vi "LX-runtime.vi"(11 "Start Time 2":u32) -> (3 "运行时间 2":dbl)   [LabVIEW 2017]
panel:
  out "Start Time":u32
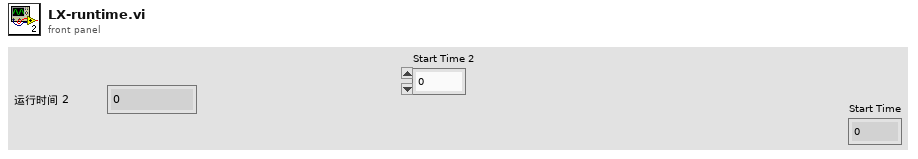
[diagram p1: front panel]
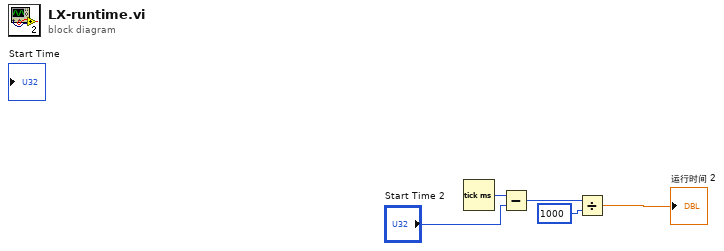
[diagram p0: block diagram]
diagram:
  n1 = Tick Count (ms)() -> (millisecond timer value=w4:u32)
  n2 = Subtract(x=w4, y="Start Time 2") -> (x-y=w5:u32)
  n3 = Divide(x=w5, y=u32 1000) -> (x/y=→"运行时间 2":dbl)
